vi "17.1.4 Classifier Evaluation.vi"() -> ()   [LabVIEW 2017]
doc: "This example shows how to use the classification VIs in NI Vision.\n\nClassification quickly identifies and classifies unknown objects in inspection images. First, use the Classification Training Interface to teach your application the types, or classes, of objects you want to classify. The Classification Training Interface creates a classifier file, which you then use to classify unknown objects into one of the classes you trained."
uses:
  <vilib>/vision/NI_Vision_Development_Module.lvlib
panel:
  out "Cross Validation Accuracy":dbl
  out "Class Predictive Value":dbl[](array[numeric]) format="%.2f"
  out "Classification Distribution":i32[][](array[numeric])
  out "Classes":string[](array[string])
  out "Class Accuracy":dbl[](array[numeric]) format="%.2f"
  out "Accuracy":sgl format="%.2f"
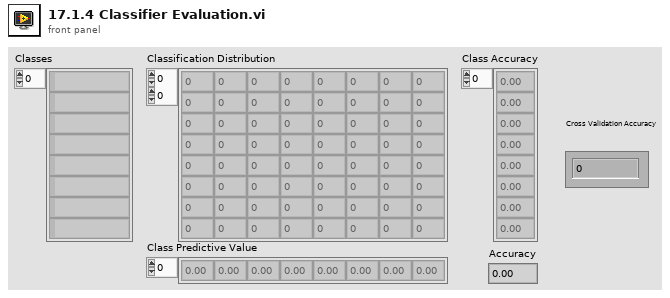
[diagram p1: front panel]
types:
  T1 = typedef "IMAQ Classifier Session.ctl" = refnum<k1>
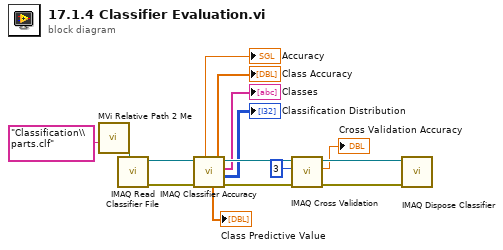
[diagram p0: block diagram]
diagram:
  n1 = call "MVi Relative Path 2 Me.vi"("Relative Path"="Classification\\parts.clf" ("name or relative path")) -> ("Appended Dir"=w14:path)  [unwired: 5 in, 1 out]
  n2 = call "IMAQ Read Classifier File"("File Path"=w14) -> ("error out"=w10:errorcluster, "Classifier Session"=w13:T1)  [unwired: 3 in, 6 out]
  n3 = call "IMAQ Classifier Accuracy"("error in (no error)"=w10, "Classifier Session"=w13) -> ("error out"=w9:errorcluster, "Classification Distribution"=→"Classification Distribution":i32[][], "Classes"=→"Classes":string[], "Classifier Session (dup)"=w12:T1, "Class Predictive Value"=→"Class Predictive Value":dbl[], "Class Accuracy"=→"Class Accuracy":dbl[], "Accuracy"=→"Accuracy":sgl)  [unwired: 3 in]
  n4 = call "IMAQ Cross Validation"("error in (no error)"=w9, "K - Value"=u32 3, "Classifier Session"=w12) -> ("error out"=w8:errorcluster, "Cross Validation Accuracy"=→"Cross Validation Accuracy":dbl, "Classifier Session (dup)"=w11:T1)  [unwired: 4 in]
  n5 = call "IMAQ Dispose Classifier"("error in (no error)"=w8, "Classifier Session"=w11) -> ()  [unwired: 10 out]
